vi "test_Create Message Group_Message Group created with desired Name.vi"(8 "error in (no error)":errorcluster, 11 "TestCase in":refnum<class "Instrument Addon Scripting API Messages Unit Tests.lvclass">) -> (0 "error out":errorcluster, 3 "TestCase out":refnum<class "Instrument Addon Scripting API Messages Unit Tests.lvclass">)   [LabVIEW 2019, in "Instrument Addon Scripting API Messages Unit Tests.lvclass"]
uses:
  Instrument Addon Scripting API Messages Unit Tests.lvclass
  <vilib>/addons/_JKI Toolkits/VI Tester/TestCase.llb/TestCase.lvclass
  Addon/Addon Shared/SubVIs/Constants.vi
  Addon/Addon Shared/Instrument Addon Shared.lvlib
  NationalInstruments.VeriStand.SystemDefinitionAPI
  <vilib>/NI VeriStand/Custom Device API/Custom Device API.lvlib
  APIs/Scripting API/Instrument Addon Scripting API.lvlib
  Instrument Addon Scripting API Test Assets/Instrument Addon Scripting API Test Assets.lvclass
  C:/Program Files (x86)/National Instruments/LabVIEW 2018/vi.lib/addons/_JKI Toolkits/VI Tester/TestCase.llb/TestCase.lvclass
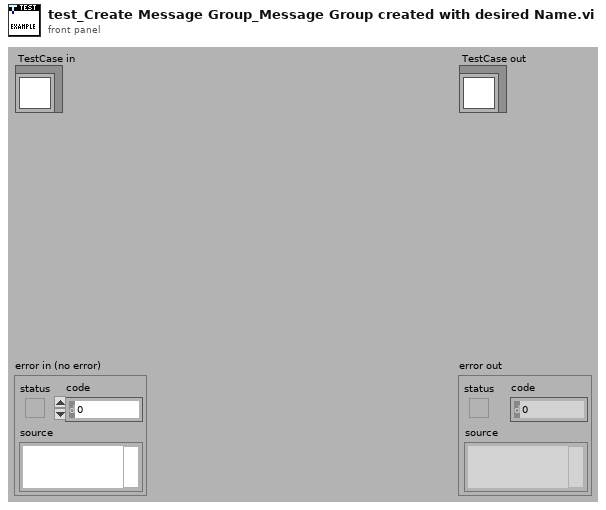
[diagram p1: front panel]
types:
  T1 = typedef "Custom Device API.lvlib/Custom Device Item Ref.ctl" = u64
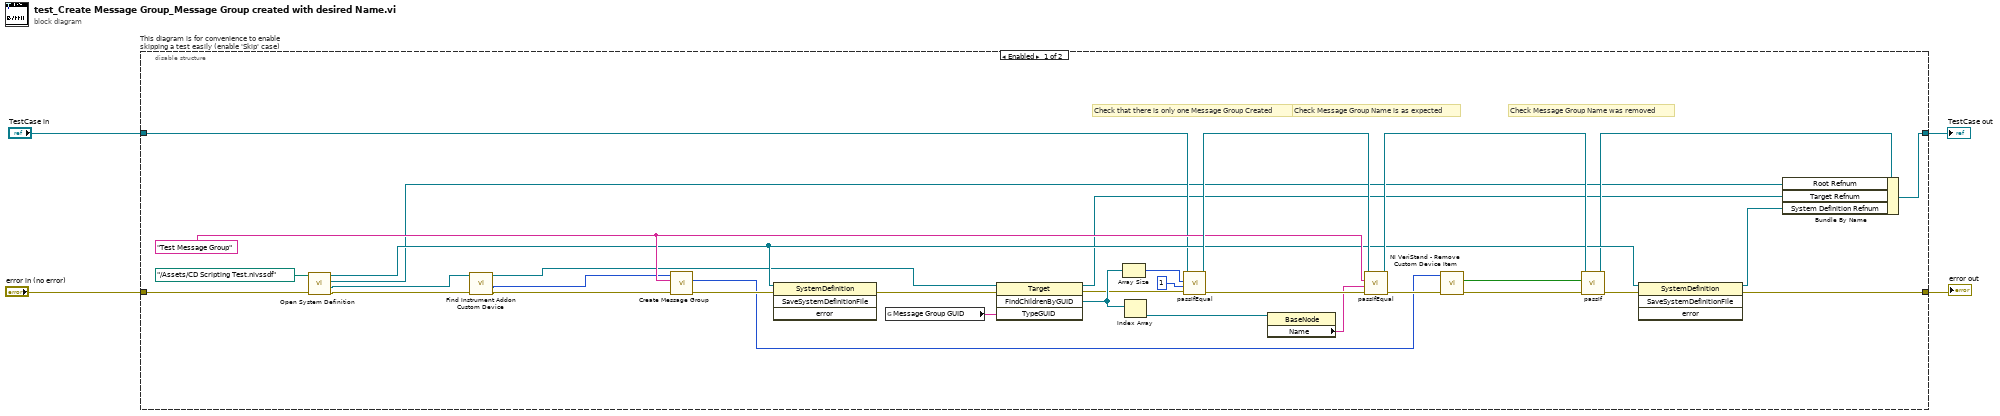
[diagram p0: block diagram]
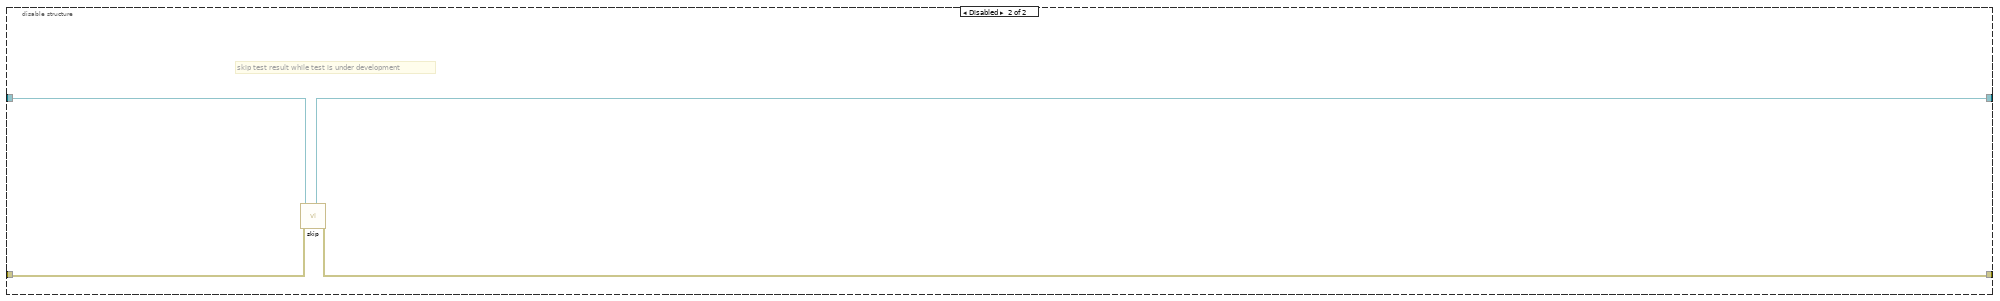
[diagram p2: hidden frame]
diagram:
  n1 = disable-structure "This diagram is for convenience to enable skipping a test easily (enable 'Skip' case)" shown="Enabled" {
    disable-tunnel: "TestCase in" -> [w10 w41]
    disable-tunnel: [w7 w39] -> w1
    disable-tunnel: [w11 w40] -> w3
    disable-tunnel: "error in (no error)" -> [w20 w38]
    frame Enabled {
      w24 = "Test Message Group" ("Section Name")
      # "Check Message Group Name was removed"
      # "Check Message Group Name is as expected"
      # "Check that there is only one Message Group Created"
      n2 = call "Open System Definition.vi"("error in (no error)"=w20, "System Definition File"=path "../Assets/CD Scripting Test.nivssdf" ("SDF file")) -> ("error out"=w16:errorcluster, "Target Refnum"=w17:refnum<k24>, "Root Refnum"=w5:refnum<k24>, "System Definition Refnum"=w18:refnum<k24>)  [unwired: 6 in]
      n3 = call "Find Instrument Addon Custom Device.vi"("error in"=w16, "target in"=w17) -> ("error out"=w13:errorcluster, "NodeID"=w14:u64, "target out"=w15:refnum<k24>)  [unwired: 7 in]
      n4 = call "Create Message Group.vi"("error in (no error)"=w13, "message group name"=w24, "instrument addon refnum in"=w14) -> ("error out"=w23:errorcluster, "message group refnum out"=w21:T1)  [unwired: 6 in, 1 out]
      n5 = invoke class="SystemDefinition" method="SaveSystemDefinitionFile"(reference=w18, error in=w23) -> (error out=w22:errorcluster)  [unwired: 2 in, 3 out]
      n6 = global read "Constants.vi" "Message Group GUID"() -> (w37:string)
      n7 = invoke class="Target" method="FindChildrenByGUID"(reference=w15, error in=w22, "TypeGUID"=w37) -> (reference out=w6:refnum<k24>, error out=w12:errorcluster, "FindChildrenByGUID"=w36:refnum<k24>[])  [unwired: 1 in, 1 out]
      n8 = Array Size(array=w36) -> (size(s)=w35:i32)
      n9 = Index Array(array=w36) -> (element=w30:refnum<k24>)  [unwired: 1 in]
      n10 = call-dynamic "passIfEqual.vi"("error in (no error)"=w12, "y"=1 ("size(s)"), "x"=w35, "TestCase in"=w10) -> ("error out"=w33:errorcluster, "TestCase out"=w32:refnum<class "Instrument Addon Scripting API Messages Unit Tests.lvclass">)  [unwired: 6 in]
      n11 = property class="BaseNode"(reference=w30) -> ("Name"=w31:string)  [unwired: 1 in, 2 out]
      n12 = call-dynamic "passIfEqual.vi"("error in (no error)"=w33, "y"=w31, "x"=w24, "TestCase in"=w32) -> ("error out"=w29:errorcluster, "TestCase out"=w25:refnum<class "Instrument Addon Scripting API Messages Unit Tests.lvclass">)  [unwired: 6 in]
      n13 = call <vilib>:"NI VeriStand - Remove Custom Device Item.vi"("error in (no error)"=w29, "Item Ref in"=w21) -> ("error out"=w28:errorcluster, "Deleted?"=w26:bool)  [unwired: 8 in]
      n14 = call-dynamic "passIf.vi"("error in (no error)"=w28, "pass"=w26, "TestCase in"=w25) -> ("error out"=w27:errorcluster, "TestCase out"=w8:refnum<class "Instrument Addon Scripting API Messages Unit Tests.lvclass">)  [unwired: 7 in]
      n15 = invoke class="SystemDefinition" method="SaveSystemDefinitionFile"(reference=w18, error in=w27) -> (reference out=w9:refnum<k24>, error out=w11:errorcluster)  [unwired: 2 in, 2 out]
      n16 = Bundle By Name(cluster=w8, "Root Refnum"=w5, "Target Refnum"=w6, "System Definition Refnum"=w9) -> (w7:refnum<class "Instrument Addon Scripting API Messages Unit Tests.lvclass">)
    }
    frame Disabled {
      # "skip test result while test is under development"
      n17 = call <vilib>:"skip.vi"("error in (no error)"=w38, "TestCase in"=w41) -> ("error out"=w40:errorcluster, "TestCase out"=w39:refnum<class "Instrument Addon Scripting API Messages Unit Tests.lvclass">)  [unwired: 8 in]
    }
  }
  "error out" <- w3
  "TestCase out" <- w1
